vi "Hardware-Phase2SensorsOutputCalPoints.vi"(4 "UEGO Diagnostics":T3={"UEGO1SensorFault"=63, "UEGO2SensorFault"=63, "UEGO1HeaterFault"=192, "UEGO2HeaterFault"=192, "UEGOFuseStatus"=0, "Battery (V)"=0.0, "LSUType"=0} {"LSUType" items=["LSU 4.9", "LSU 4.2"]; "UEGOFuseStatus" items=["FUSE OK", "FUSE BLOWN"]; "UEGO2SensorFault" items=["NO FAULT"=63, "SHORT TO GND OR BATT"=0]; "UEGO2HeaterFault" items=["SHORT TO GROUND"=0, "OPEN CIRCUIT"=64, "SHORT TO BATTERY"=128, "NO FAULT"=192]; "UEGO1SensorFault" items=["NO FAULT"=63, "SHORT TO GND OR BATT"=0]; "UEGO1HeaterFault" items=["SHORT TO GROUND"=0, "OPEN CIRCUIT"=64, "SHORT TO BATTERY"=128, "NO FAULT"=192]}, 5 "UEGO Temperature":T2, 6 "UEGO Sensor Results":T1) -> ()   [LabVIEW 2015, in "DSI-RT.lvlib"]
uses:
  DSI-RT.lvlib
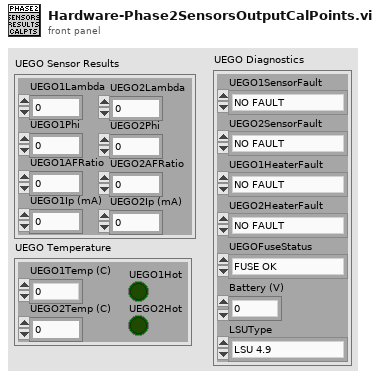
[diagram p1: front panel]
types:
  T1 = cluster{"UEGO1Lambda":sgl, "UEGO1Phi":sgl, "UEGO1AFRatio":sgl, "UEGO1Ip (mA)":sgl, "UEGO2Lambda":sgl, "UEGO2Phi":sgl, "UEGO2AFRatio":sgl, "UEGO2Ip (mA)":sgl}
  T2 = cluster{"UEGO1Temp (C)":sgl, "UEGO2Temp (C)":sgl, "UEGO1Hot":bool, "UEGO2Hot":bool}
  T3 = cluster{"UEGO1SensorFault":u8, "UEGO2SensorFault":u8, "UEGO1HeaterFault":u8, "UEGO2HeaterFault":u8, "UEGOFuseStatus":u8, "Battery (V)":sgl, "LSUType":u8}
  T4 = cluster{"UEGO1SensorFault":sgl, "UEGO2SensorFault":sgl, "UEGO1HeaterFault":sgl, "UEGO2HeaterFault":sgl, "UEGOFuseStatus":sgl, "Battery (V)":sgl, "LSUType":sgl}
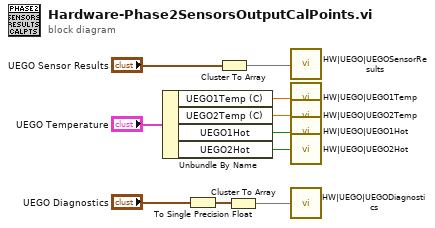
[diagram p0: block diagram]
diagram:
  n1 = Unbundle By Name("UEGO Temperature") -> ("UEGO1Temp (C)"=w8:sgl, "UEGO2Temp (C)"=w7:sgl, "UEGO1Hot"=w6:bool, "UEGO2Hot"=w5:bool)
  n2 = To Single Precision Float(number="UEGO Diagnostics") -> (single precision float=w3:T4)
  n3 = Cluster To Array(cluster="UEGO Sensor Results") -> (array=w9:sgl[])
  n4 = Cluster To Array(cluster=w3) -> (array=w1:sgl[])
  n5 = call "HW|UEGO|UEGOSensorResults"("Value"=w9) -> ()
  n6 = call "HW|UEGO|UEGO1Temp"("Value"=w8) -> ()
  n7 = call "HW|UEGO|UEGO2Temp"("Value"=w7) -> ()
  n8 = call "HW|UEGO|UEGO1Hot"("Value"=w6) -> ()
  n9 = call "HW|UEGO|UEGO2Hot"("Value"=w5) -> ()
  n10 = call "HW|UEGO|UEGODiagnostics"("Value"=w1) -> ()
